vi "Drive Controller.vi"(8 "error in":errorcluster) -> ()   [LabVIEW 2015]
doc: "This VI executes continuously carrying out the current operation and responding to updates or new operation requests. It will often contain the timing or control code that is difficult to place directly in TeleOp. This VI generally opens all sensors and motors and isolates the rest of the robot code from knowing implementation details of how the operations are carried out."
uses:
  Drive Setpoints.ctl
  Drive Operations.ctl
  <vilib>/Rock Robotics/WPI/SafetyOutput/WPI_SafetyOutputConfigMenu.ctl
  <vilib>/Rock Robotics/WPI/CAN/TalonSRX/WPI_CANTalonSRX_APIControlMode.ctl
panel:
  in  "Numeric":dbl
  out "Setpoints":T1(graph)
  out "Current\nCmd":string
  # "Tip: It may be helpful to observe inputs and sensor values.\nYou may also want to display tuning or debugging controls."
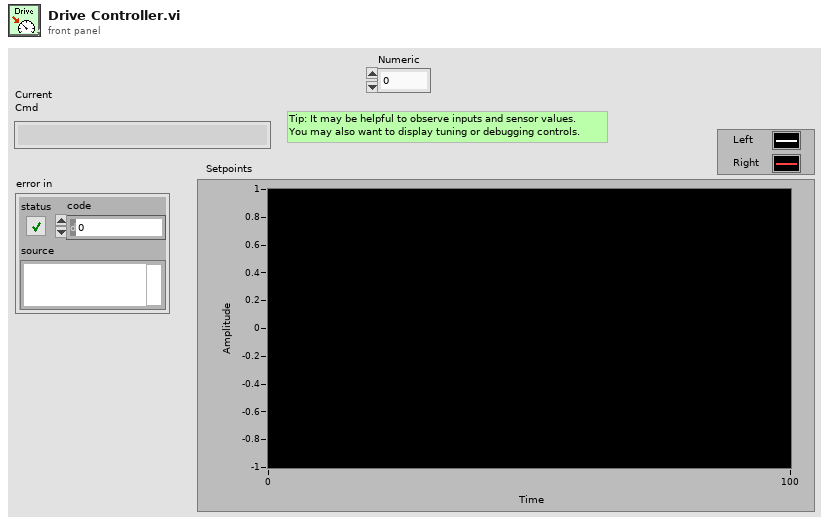
[diagram p1: front panel]
types:
  T1 = cluster{"Left Setpoint":dbl, "Right Setpoint":dbl}
  T2 = typedef "WPI_CANTalonSRX_APIControlMode.ctl" = enum8{"Percent VBus", "Speed", "Position", "Slave", "Unchanged / Invalid", "Voltage Compensation", "Current", "Motion Profile"}
  T3 = typedef "WPI_SafetyOutputConfigMenu.ctl" = enum16{"Enable", "Disable"}
  T4 = typedef "Drive Setpoints.ctl" = cluster{"Operation":T5, "Left Setpoint":dbl, "Right Setpoint":dbl, "Duration":dbl}
  T5 = typedef "Drive Operations.ctl" = enum16{"Reserve", "Read Current", "Immediate", "Drive for Time", "Drive for Distance"}
  T6 = typedef "WPI_MotorControlDeviceRef.ctl" = cluster{"DeviceStatus":errorcluster, "Type":T7, "PWM":cluster{"PWM Channel":T8, "DeadBand":T9}, "CAN":cluster{"Device Number":u8, "Control Mode":T10, "Semaphore":T11, "Max Vout":dbl, "TalonSRX Control Mode":T2}, "Invert":bool}
  T7 = typedef "WPI_MotorControlType.ctl" = enum16{"PWM", "CAN", "CANTalonSRX"}
  T8 = typedef "FPGA_DIOPWMChannel.ctl" = enum8{"PWM 0", "PWM 1", "PWM 2", "PWM 3", "PWM 4", "PWM 5", "PWM 6", "PWM 7", "PWM 8", "PWM 9", "PWM MXP 0", "PWM MXP 1", "PWM MXP 2", "PWM MXP 3", "PWM MXP 4", "PWM MXP 5", "PWM MXP 6", "PWM MXP 7", "PWM MXP 8", "PWM MXP 9", "Invalid"}
  T9 = typedef "WPI_PWMDeadband.ctl" = cluster{"Name":string, "maxPositivePwm":i32, "minPositivePwm":i32, "centerPwm":i32, "maxNegativePwm":i32, "minNegativePwm":i32, "angularRange":u16}
  T10 = typedef "WPI_CANJaguar_ControlMode.ctl" = enum8{"Percent VBus", "Current", "Speed", "Position", "Voltage"}
  T11 = typedef "Semaphore RefNum" = refnum<k1>
  T12 = typedef "WPI_RobotDriveDevRef.ctl" = cluster{"DevStatus":errorcluster, "Motors[]":T6[], "Square Inputs":bool, "Max Output":dbl}
  T13 = typedef "Command Status Info.ctl" = cluster{"Name":string, "Status":T14, "notifier out":T15}
  T14 = typedef "Completion Status.ctl" = enum16{"Successful", "Aborted", "Incomplete"}
  T15 = typedef "Completion Notifier.ctl" = refnum<notifier>
  T16 = cluster{"SubSystem Data":T4, cluster{"Start Time (ms)":u32, "Iterations":i32}, cluster{"Command Info":T13, "Description":string, "SubSystem Data":T4, "notifier out":refnum<notifier>, "Subsystem Name":string}}
  T17 = cluster{"SubSystem Data":T4, cluster{"Start Time (ms)":u32, "Iterations":i32}, "Default Command Arguments":cluster{"Command Info":T13, "Description":string, "SubSystem Data":T4, "notifier out":refnum<notifier>, "Subsystem Name":string}}
  T18 = cluster{"Don't move motors while reserved":dbl, "Don't move motors while reserved":dbl}
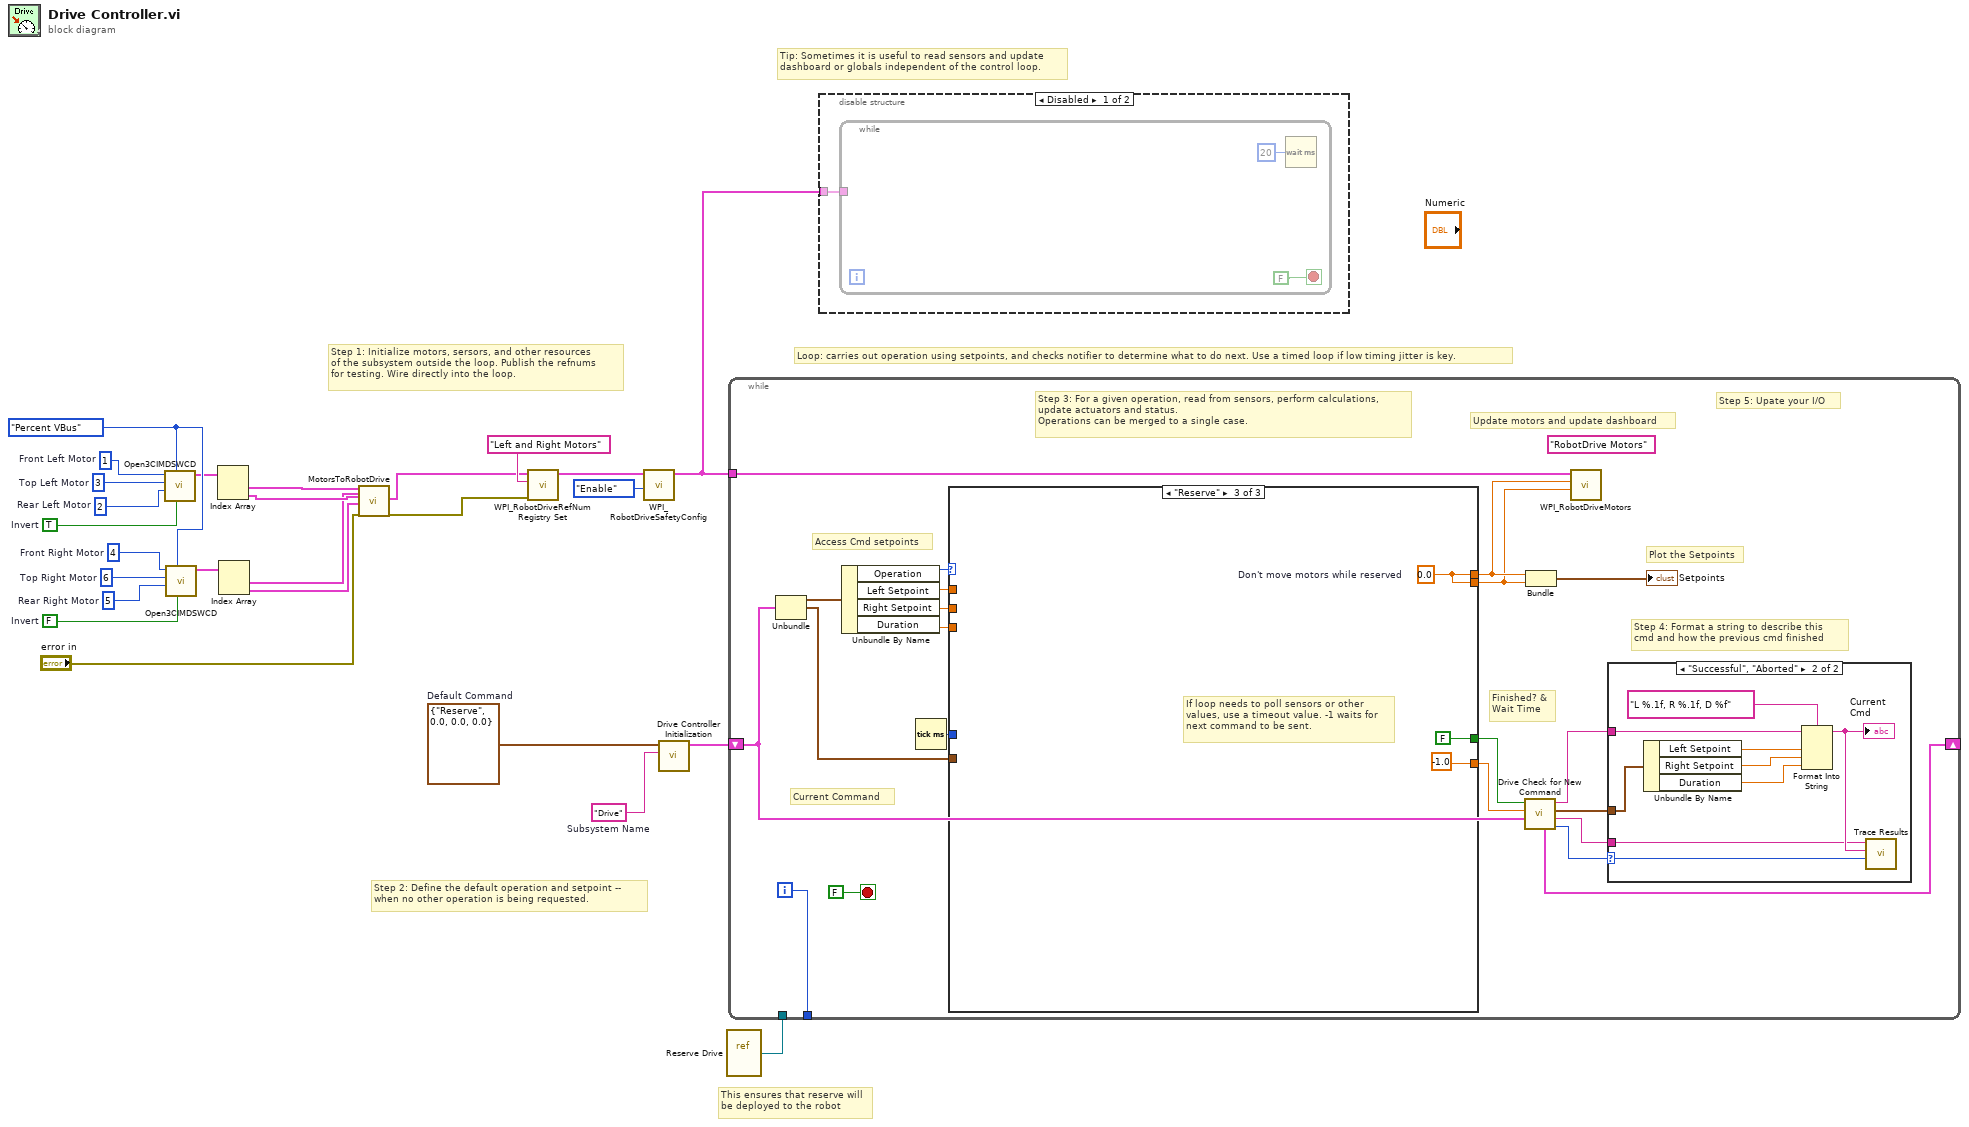
[diagram p0: block diagram]
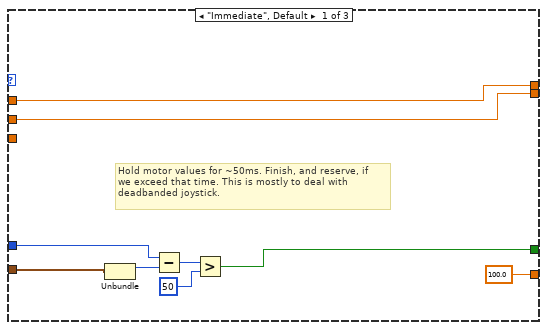
[diagram p4: hidden frame]
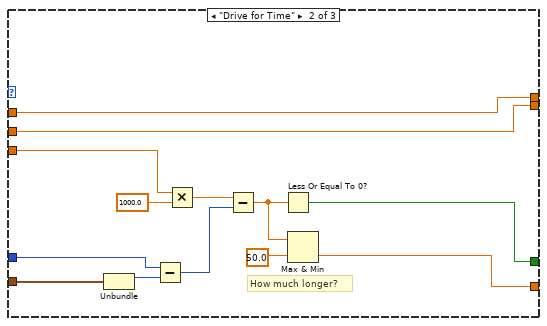
[diagram p5: hidden frame]
diagram:
  w10 = FALSE  # Invert
  w15 = TRUE  # Invert
  w12 = u8 6  # Top Right Motor
  w11 = u8 5  # Rear Right Motor
  w13 = u8 4  # Front Right Motor
  w17 = u8 3  # Top Left Motor
  w16 = u8 2  # Rear Left Motor
  w18 = u8 1  # Front Left Motor
  w14 = WPI_CANTalonSRX_APIControlMode."Percent VBus" ("Control Mode")
  w25 = T4 {"Operation"=enum."Reserve", "Left Setpoint"=0.0, "Right Setpoint"=0.0, "Duration"=0.0}  # Default Command
  w26 = "Drive"  # Subsystem Name
  # "This ensures that reserve will\nbe deployed to the robot"
  # "Tip: Sometimes it is useful to read sensors and update\ndashboard or globals independent of the control loop."
  # "Step 2: Define the default operation and setpoint --\nwhen no other operation is being requested."
  # "Step 1: Initialize motors, sersors, and other resources\nof the subsystem outside the loop. Publish the refnums\nfor testing. Wire directly into the loop."
  # "Loop: carries out operation using setpoints, and checks notifier to determine what to do next. Use a timed loop if low timing jitter is key."
  n1 = call "Open3CIMDSWCD.vi"("Invert"=w15, "Control Mode"=w14, "Bottom Back"=w16, "Top Middle"=w17, "Bottom Front"=w18) -> ("Motor Instances"=w9:T6[])  [unwired: 6 in]
  n2 = call "Open3CIMDSWCD.vi"("Invert"=w10, "Control Mode"=w14, "Bottom Back"=w11, "Top Middle"=w12, "Bottom Front"=w13) -> ("Motor Instances"=w6:T6[])  [unwired: 6 in]
  n3 = Index Array(array=w9) -> (element #1=w8:T6, element #2=w7:T6)  [unwired: 2 in]
  n4 = Index Array(array=w6) -> (element #1=w5:T6, element #2=w4:T6)  [unwired: 2 in]
  n5 = call "MotorsToRobotDrive.vi"("Left Motor 1"=w8, "Right Motor 1"=w5, "Left Motor 2"=w7, "Right Motor 2"=w4, "error in"="error in") -> ("RobotDriveDevRef"=w3:T12, "error out"=w2:errorcluster)  [unwired: 13 in]
  n6 = call <vilib>:"WPI_RobotDriveRefNum Registry Set.vi"("error in (no error)"=w2, "refnum name"="Left and Right Motors", "RobotDriveDevRef"=w3) -> ("RobotDriveDevRef"=w23:T12)  [unwired: 1 in, 7 out]
  n7 = call <vilib>:"WPI_RobotDriveSafetyConfig.vi"("mode"=WPI_SafetyOutputConfigMenu."Enable", "RobotDriveDevRef"=w23) -> ("RobotDriveDevRef"=w21:T12)  [unwired: 8 in, 1 out]
  n8 = call "Drive Controller Initialization.vi"("Subsystem Name"=w26, "Default Command"=w25) -> ("output cluster"=w20:T16)  [unwired: 9 in]
  n9 = vi-ref "Reserve Drive.vi"() -> (w19:refnum<vi>)
  n10 = while {
    shift-right: [w34] -> _
    shift-left: w20 -> [w27]
    tunnel: [w46] -> _
    tunnel: w21 -> [w42]
    tunnel: w19 -> [_]
    i -> [w46]
    stop <- FALSE stop-if-true
    (unwired) "RobotDrive Motors" ("Name")
    # "Step 5: Upate your I/O"
    # "Step 4: Format a string to describe this\ncmd and how the previous cmd finished"
    # "Current Command"
    # "Update motors and update dashboard"
    # "Plot the Setpoints"
    # "Access Cmd setpoints"
    # "Finished? &\nWait Time"
    # "Step 3: For a given operation, read from sensors, perform calculations,\nupdate actuators and status.\nOperations can be merged to a single case."
    n11 = Unbundle(w27) -> ("SubSystem Data"=w41:T4, w28:cluster{"Start Time (ms)":u32, "Iterations":i32})  [unwired: 1 out]
    n12 = Unbundle By Name(w41) -> ("Operation"=w40:T5, "Left Setpoint"=w39:dbl, "Right Setpoint"=w38:dbl, "Duration"=w37:dbl)
    n13 = Tick Count (ms)() -> (millisecond timer value=w36:u32)
    n14 = case shown="\"Reserve\"" w40 {
      tunnel: [100.0 w66 -1.0] -> w33
      tunnel: [w58 w73 FALSE ("ignore previous (F)")] -> w32
      tunnel: w28 -> [w57 w75 _]
      tunnel: [w64 w72 w79] -> w44
      tunnel: [w63 w71 w79] -> w43
      tunnel: w39 -> [w64 w72 _]
      tunnel: w38 -> [w63 w71 _]
      tunnel: w37 -> [_ w70 _]
      tunnel: w36 -> [w59 w69 _]
      frame "Immediate", Default {
        # "Hold motor values for ~50ms. Finish, and reserve, if\nwe exceed that time. This is mostly to deal with\ndeadbanded joystick."
        n15 = Unbundle(w57) -> ("Start Time (ms)"=w60:u32)  [unwired: 1 out]
        n16 = Subtract(x=w59, y=w60) -> (x-y=w61:u32)
        n17 = Greater?(x=w61, y=u8 50 ("Left Motor")) -> (0:w58:bool)
      }
      frame "Drive for Time" {
        # "How much longer?"
        n18 = Unbundle(w75) -> ("Start Time (ms)"=w74:u32)  [unwired: 1 out]
        n19 = Subtract(x=w69, y=w74) -> (x-y=w78:u32)
        n20 = Multiply(x=w70, y=1000.0) -> (x*y=w77:dbl)
        n21 = Subtract(x=w77, y=w78) -> (x-y=w68:dbl)
        n22 = Less Or Equal To 0?(x=w68) -> (x <= 0?=w73:bool)
        n23 = Max & Min(x=w68, y=50.0) -> (min(x,y)=w66:dbl)  [unwired: 1 out]
      }
      frame "Reserve" {
        w79 = 0.0  # Don't move motors while reserved
        # "If loop needs to poll sensors or other\nvalues, use a timeout value. -1 waits for\nnext command to be sent."
      }
    }
    n24 = call "Drive Check for New Command.vi"("input cluster"=w27, "Wait time (ms)"=w33, "Finished?"=w32) -> ("Completion"=w35:T14, "Subsystem Name"=w29:string, "SetPoint"=w30:T4, "Initial Trace String"=w31:string, "output cluster"=w34:T17)  [unwired: 4 in]
    n25 = Bundle("Don't move motors while reserved"=w44, "Don't move motors while reserved"=w43) -> (→"Setpoints":T18)  [unwired: 1 in]
    n26 = call <vilib>:"WPI_RobotDriveMotors.vi"("RightSpeed"=w43, "LeftSpeed"=w44, "RobotDriveDevRef"=w42) -> ()  [unwired: 1 in, 8 out]
    n27 = case shown="\"Successful\", \"Aborted\"" w35 {
      selector: w35 -> [_ w56]
      tunnel: w31 -> [_ w51]
      tunnel: w30 -> [_ w52]
      tunnel: w29 -> [_ w48]
      frame "Incomplete", Default {
        # "Continuing current command"
      }
      frame "Successful", "Aborted" {
        # "Report and setup for next command"
        n28 = Unbundle By Name(w52) -> ("Left Setpoint"=w54:dbl, "Right Setpoint"=w55:dbl, "Duration"=w49:dbl)
        n29 = Format Into String(format string="L %.1f, R %.1f, D %f", initial string=w51, w54, w55, w49) -> (resulting string=w50:string)  [unwired: 1 in, 1 out]
        "Current\nCmd" <- w50
        n30 = call <vilib>:"Trace Results.vi"("Status of previous command"=w56, "Description"=w50, "Subsystem"=w48) -> ()  [unwired: 9 in]
      }
    }
  }
  n31 = disable-structure shown="Disabled" {
    disable-tunnel: w21 -> [w82 _]
    frame Disabled {
      n32 = while {
        tunnel: w82 -> [_]
        stop <- FALSE stop-if-true
        n33 = Wait (ms)(milliseconds to wait=u32 20) -> ()  [unwired: 1 out]
      }
    }
    frame Enabled {
    }
  }
